vi "Camera Setup.vi"(11 "SceneGraphDisplay in":refnum<vi>) -> (0 "error out":errorcluster)   [LabVIEW 2013]
uses:
  <vilib>/Utility/miscctls.llb/LV3DPointTypeDef.ctl
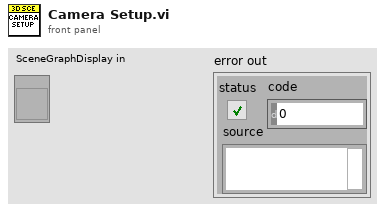
[diagram p1: front panel]
types:
  T1 = typedef "LV3DPointTypeDef.ctl" = cluster{"X":sgl, "Y":sgl, "Z":sgl}
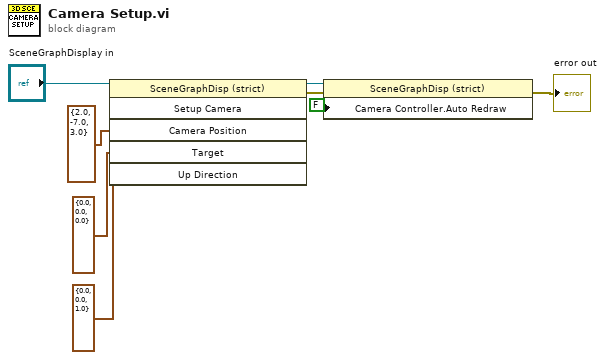
[diagram p0: block diagram]
diagram:
  n1 = invoke on="Invoke Node" class="SceneGraphDisp (strict)" method="Setup Camera"(reference="SceneGraphDisplay in", "Camera Position"=T1 {"X"=2.0, "Y"=-7.0, "Z"=3.0}, "Target"=T1 {"X"=0.0, "Y"=0.0, "Z"=0.0}, "Up Direction"=T1 {"X"=0.0, "Y"=0.0, "Z"=1.0}) -> (reference out=w5:refnum<vi>, error out=w6:errorcluster)  [unwired: 2 in, 4 out]
  n2 = property on="Property Node" class="SceneGraphDisp (strict)"(reference=w5, error in=w6, "Camera Controller.Auto Redraw"=FALSE ("Camera Controller:Auto Redraw")) -> (error out=→"error out":errorcluster)  [unwired: 1 out]
